vi "http transmit response.vi"(8 "error in":errorcluster, 10 "application request":T1, 11 "tcp connection":refnum<k5>) -> (0 "error out":errorcluster)   [LabVIEW 2016, in "Basic HTTP server.lvclass"]
uses:
  Basic HTTP server.lvclass
  http response.ctl
  http response packet type.ctl
  HTTP headers/http header data.ctl
  HTTP headers/http headers.lvlib
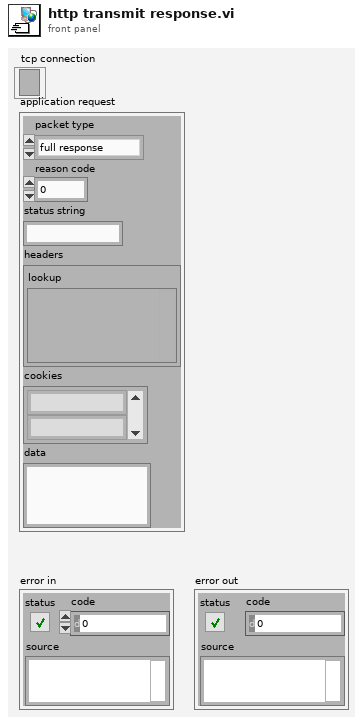
[diagram p1: front panel]
types:
  T1 = typedef "Basic HTTP server.lvclass/http response.ctl" = cluster{"packet type":T2, "reason code":u16, "status string":string, "headers":T3, "cookies":string[], "data":string}
  T2 = typedef "Basic HTTP server.lvclass/http response packet type.ctl" = enum16{"full response", "header only", "data only", "last data", "raw output"}
  T3 = typedef "http headers.lvlib/http header data.ctl" = cluster{"lookup":variant}
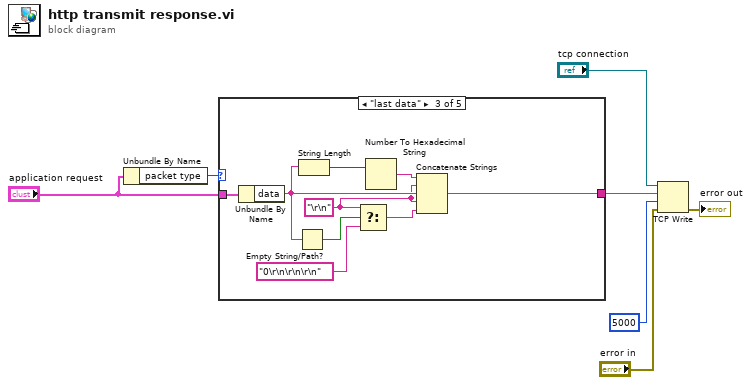
[diagram p0: block diagram]
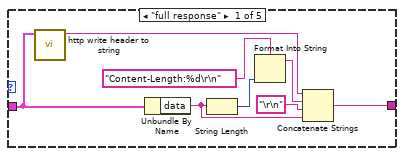
[diagram p2: hidden frame]
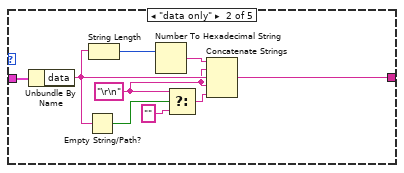
[diagram p3: hidden frame]
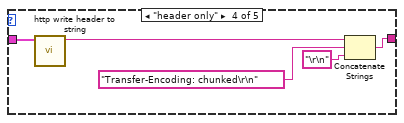
[diagram p4: hidden frame]
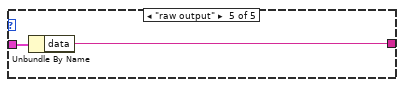
[diagram p5: hidden frame]
diagram:
  n1 = Unbundle By Name("application request") -> ("packet type"=w6:T2)
  n2 = case shown="\"last data\"" w6 {
    tunnel: "application request" -> [w10 w24 w33 w36 w40]
    tunnel: [w8 w16 w25 w34 w39] -> w1
    frame "full response" {
      n3 = call "http write header to string.vi"("application request"=w10) -> ("header string"=w9:string)  [unwired: 10 in]
      n4 = Unbundle By Name(w10) -> ("data"=w11:string)
      n5 = String Length(string=w11) -> (length=w15:i32)
      n6 = Format Into String(format string="Content-Length:%d\r\n", w15) -> (resulting string=w13:string)  [unwired: 2 in, 1 out]
      n7 = Concatenate Strings(w9, w13, "\r\n" ("format string"), w11) -> (w8:string)
    }
    frame "data only" {
      w19 = "\r\n" ("format string")
      n8 = Unbundle By Name(w24) -> ("data"=w21:string)
      n9 = Empty String/Path?(string/path=w21) -> (empty?=w20:bool)
      n10 = String Length(string=w21) -> (length=w23:i32)
      n11 = Number To Hexadecimal String(2:w23) -> (0:w22:string)  [unwired: 1 in]
      n12 = Select(t=w19, s=w20, f="") -> (s? t:f=w18:string)
      n13 = Concatenate Strings(w22, w19, w21, w19, w18) -> (w16:string)
    }
    frame "last data" {
      w28 = "\r\n" ("format string")
      n14 = Unbundle By Name(w33) -> ("data"=w30:string)
      n15 = Empty String/Path?(string/path=w30) -> (empty?=w29:bool)
      n16 = String Length(string=w30) -> (length=w31:i32)
      n17 = Select(t=w28, s=w29, f="0\r\n\r\n\r\n" ("data in")) -> (s? t:f=w26:string)
      n18 = Number To Hexadecimal String(2:w31) -> (0:w32:string)  [unwired: 1 in]
      n19 = Concatenate Strings(w32, w28, w30, w28, w26) -> (w25:string)
    }
    frame "header only" {
      n20 = call "http write header to string.vi"("application request"=w36) -> ("header string"=w35:string)  [unwired: 10 in]
      n21 = Concatenate Strings(w35, "Transfer-Encoding: chunked\r\n" ("format string"), "\r\n" ("format string")) -> (w34:string)
    }
    frame "raw output" {
      n22 = Unbundle By Name(w40) -> ("data"=w39:string)
    }
  }
  n23 = TCP Write(connection ID="tcp connection", data in=w1, error in (no error)="error in", 9:5000 ("timeout ms (25000)")) -> (error out=→"error out":errorcluster)  [unwired: 2 out]
